vi "tempAndVoltage.vi"() -> ()   [LabVIEW 2018]
panel:
  in  "opsensModulePath":path=path "C:/Research/Sena's CodeBase and Documents/tempsAndScopeLabview.py"
  in  "opsensNumCollects":i32=500
  out "Opsens Channel 1":cluster{dbl[], dbl[]}(graph)
  in  "opsensReadFunction":string="opsensRead"
  out "opsensErrorOut":errorcluster
  out "Oscilloscope Channel 2 Output Graph":cluster{dbl[], dbl[]}[](graph)
  out "Oscilloscope Channel 1 Output Graph":cluster{dbl[], dbl[]}[](graph)
  in  "numChan":i32=2
  in  "scopeNumCollects":i32=2
  in  "longRecordLength 2":i32=100000
  in  "shortRecordLength":i32=10000
  in  "scopeReadFunction":string="scopeRead"
  in  "scopeModulePath":path=path "C:/Research/Sena's CodeBase and Documents/tempsAndScopeLabview.py"
  out "scopeErrorOut":errorcluster
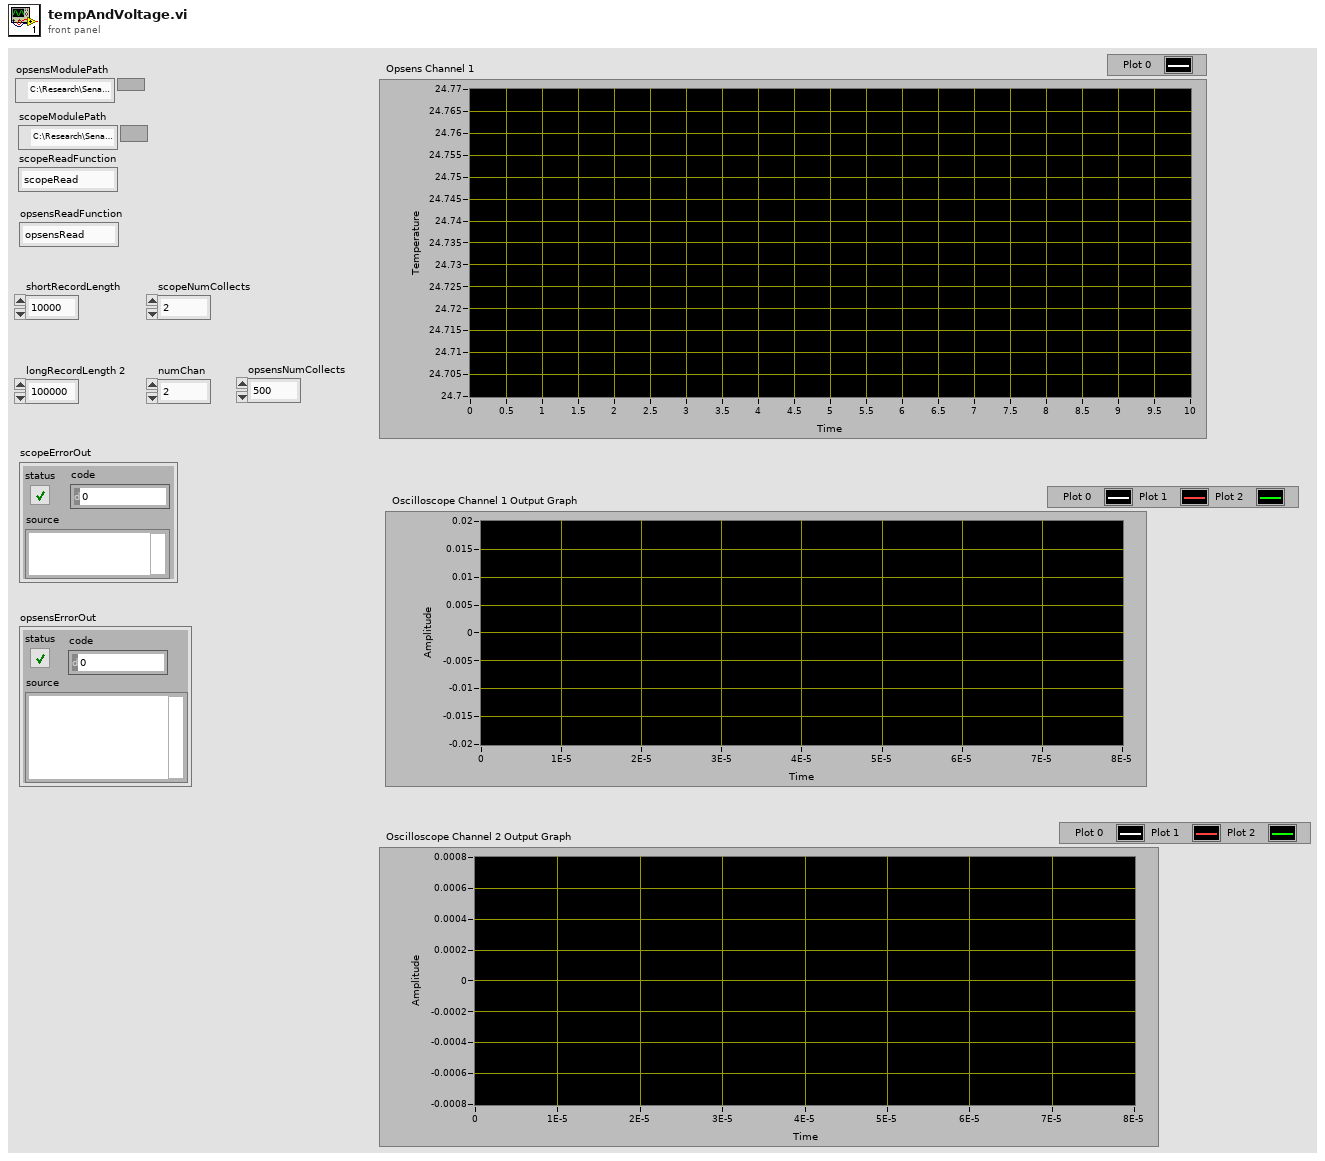
[diagram p1: front panel]
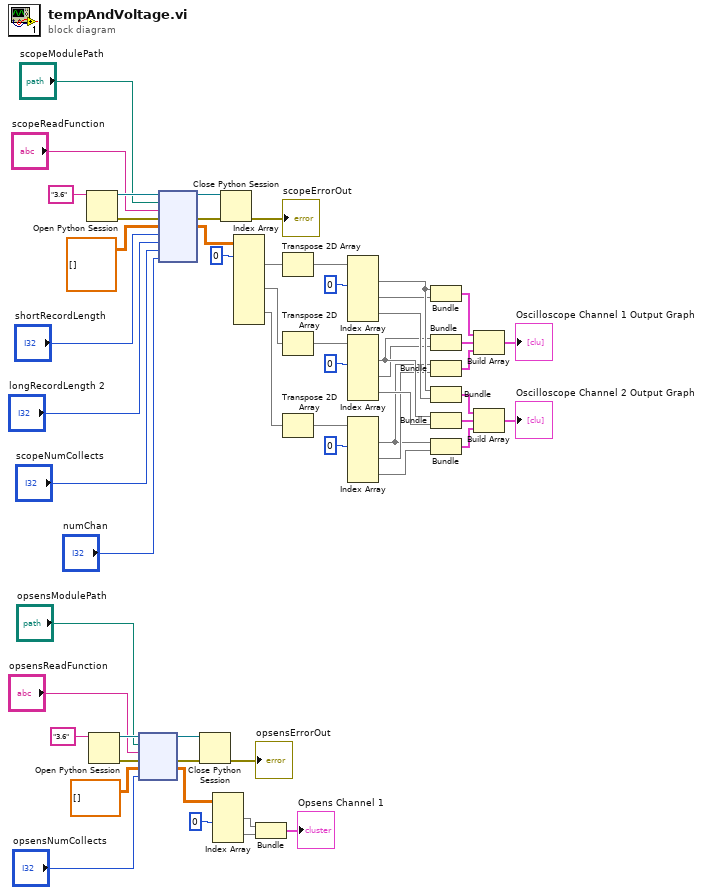
[diagram p0: block diagram]
diagram:
  n1 = Open Python Session(python version="3.6" ("Python version")) -> (session out=w56:refnum<k35>, error out=w55:errorcluster)  [unwired: 2 in]
  n2 = Open Python Session(python version="3.6") -> (session out=w15:refnum<k35>, error out=w10:errorcluster)  [unwired: 2 in]
  n3 = node(w15, "opsensModulePath", "opsensReadFunction", w10, dbl[][] [], "opsensNumCollects") -> (w14:refnum<k35>, w13:errorcluster, w4:dbl[][])  [unwired: 1 in, 2 out]
  n4 = node(w56, "scopeModulePath", "scopeReadFunction", w55, dbl[][][] [], "shortRecordLength", "longRecordLength 2", "scopeNumCollects", "numChan") -> (w37:refnum<k35>, w36:errorcluster, w47:dbl[][][])  [unwired: 4 in, 2 out]
  n5 = Close Python Session(session in=w14, error in=w13) -> (11:→"opsensErrorOut":errorcluster)
  n6 = Index Array(array=w4, index (col) #1=0 ("index")) -> (element #1=w8:dbl[], element #2=w7:dbl[])  [unwired: 3 in]
  n7 = Close Python Session(session in=w37, error in=w36) -> (11:→"scopeErrorOut":errorcluster)
  n8 = Index Array(array=w47, index (dim 0) #1=0 ("index (page)")) -> (element #1=w46:dbl[][], element #2=w43:dbl[][], element #3=w40:dbl[][])  [unwired: 8 in]
  n9 = Bundle(w8, w7) -> (→"Opsens Channel 1":cluster{dbl[], dbl[]})  [unwired: 1 in]
  n10 = Transpose 2D Array(2D array=w46) -> (transposed array=w45:dbl[][])
  n11 = Transpose 2D Array(2D array=w43) -> (transposed array=w41:dbl[][])
  n12 = Transpose 2D Array(2D array=w40) -> (transposed array=w39:dbl[][])
  n13 = Index Array(array=w45, index (col) #1=0 ("index (page)")) -> (element #1=w34:dbl[], element #2=w33:dbl[], element #3=w32:dbl[])  [unwired: 5 in]
  n14 = Index Array(array=w41, index (col) #1=0 ("index (page)")) -> (element #1=w31:dbl[], element #2=w30:dbl[], element #3=w29:dbl[])  [unwired: 5 in]
  n15 = Index Array(array=w39, index (col) #1=0 ("index (page)")) -> (element #1=w27:dbl[], element #2=w28:dbl[], element #3=w26:dbl[])  [unwired: 5 in]
  n16 = Bundle(w34, w33) -> (w24:cluster{dbl[], dbl[]})  [unwired: 1 in]
  n17 = Bundle(w31, w30) -> (w23:cluster{dbl[], dbl[]})  [unwired: 1 in]
  n18 = Bundle(w27, w28) -> (w22:cluster{dbl[], dbl[]})  [unwired: 1 in]
  n19 = Bundle(w34, w32) -> (w21:cluster{dbl[], dbl[]})  [unwired: 1 in]
  n20 = Bundle(w31, w29) -> (w20:cluster{dbl[], dbl[]})  [unwired: 1 in]
  n21 = Bundle(w27, w26) -> (w19:cluster{dbl[], dbl[]})  [unwired: 1 in]
  n22 = Build Array(w24, w23, w22) -> (→"Oscilloscope Channel 1 Output Graph":cluster{dbl[], dbl[]}[])
  n23 = Build Array(w21, w20, w19) -> (→"Oscilloscope Channel 2 Output Graph":cluster{dbl[], dbl[]}[])
